vi "Apply Container Settings.vi"(7 "Source Index":i32, 8 "error in (no error)":errorcluster, 11 "BuildSpec in":refnum<vi>) -> (0 "error out":errorcluster, 3 "BuildSpec out":refnum<vi>)   [LabVIEW 2019, in "Project Sync Tools.lvclass"]
uses:
  Project Sync Tools.lvclass
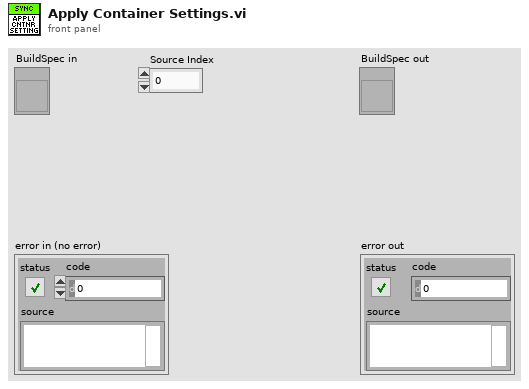
[diagram p1: front panel]
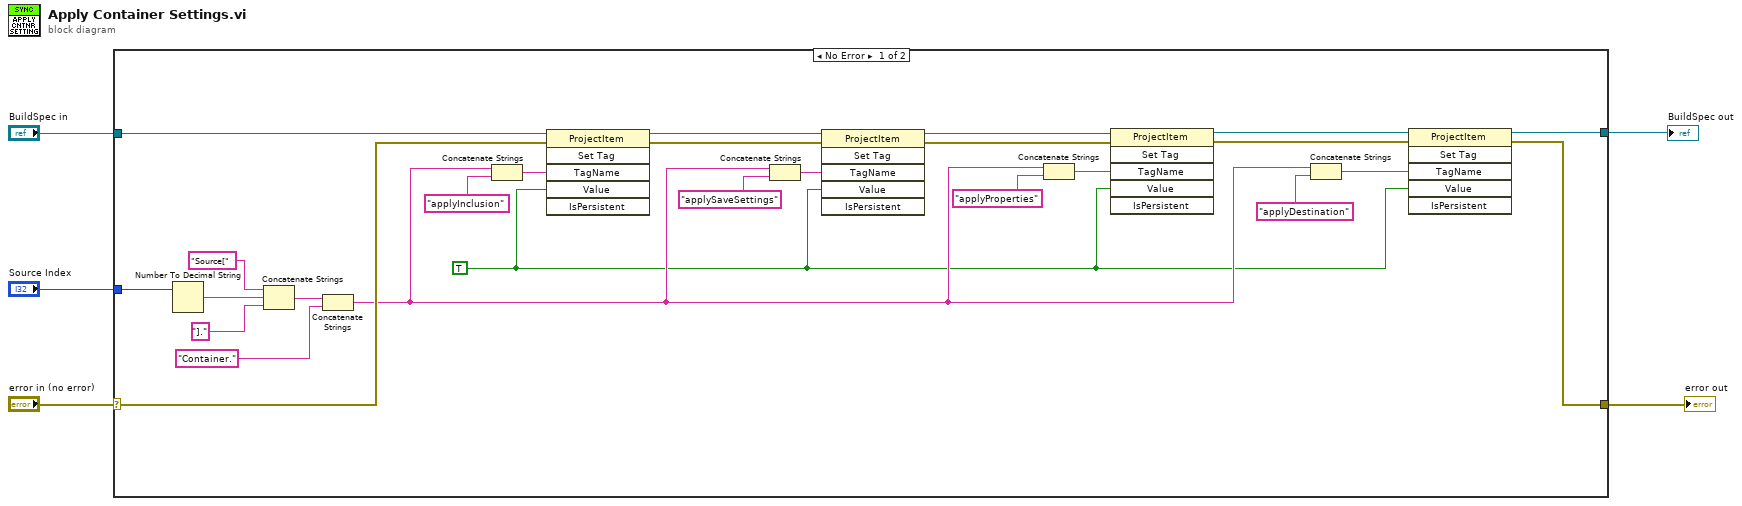
[diagram p0: block diagram]
diagram:
  n1 = case shown="No Error" "error in (no error)" {
    selector: "error in (no error)" -> [w17 w32]
    tunnel: "BuildSpec in" -> [w31 w33]
    tunnel: [w10 w32] -> w4
    tunnel: [w11 w33] -> w3
    tunnel: "Source Index" -> [w23 _]
    frame No Error {
      w6 = TRUE
      n2 = Number To Decimal String(number=w23) -> (decimal integer string=w25:string)  [unwired: 1 in]
      n3 = Concatenate Strings("Source[" ("string"), w25, "].") -> (w22:string)
      n4 = Concatenate Strings(w22, "Container." ("string")) -> (w9:string)
      n5 = Concatenate Strings(w9, "applyInclusion") -> (w14:string)
      n6 = invoke class="ProjectItem" method="Set Tag"(reference=w31, error in=w17, "TagName"=w14, "Value"=w6) -> (reference out=w27:refnum<vi>, error out=w30:errorcluster)  [unwired: 2 in, 4 out]
      n7 = Concatenate Strings(w9, "applySaveSettings") -> (w20:string)
      n8 = invoke class="ProjectItem" method="Set Tag"(reference=w27, error in=w30, "TagName"=w20, "Value"=w6) -> (reference out=w28:refnum<vi>, error out=w29:errorcluster)  [unwired: 2 in, 4 out]
      n9 = Concatenate Strings(w9, "applyProperties") -> (w18:string)
      n10 = invoke class="ProjectItem" method="Set Tag"(reference=w28, error in=w29, "TagName"=w18, "Value"=w6) -> (reference out=w13:refnum<vi>, error out=w12:errorcluster)  [unwired: 2 in, 4 out]
      n11 = Concatenate Strings(w9, "applyDestination") -> (w7:string)
      n12 = invoke class="ProjectItem" method="Set Tag"(reference=w13, error in=w12, "TagName"=w7, "Value"=w6) -> (reference out=w11:refnum<vi>, error out=w10:errorcluster)  [unwired: 2 in, 4 out]
    }
    frame Error {
    }
  }
  "error out" <- w4
  "BuildSpec out" <- w3
